vi "Read TDMS File.vi"(8 "error in (no error)":errorcluster, 11 "Path":path) -> (0 "error out":errorcluster, 2 "Data":dbl[](array[numeric]))   [LabVIEW 2022 SP3]
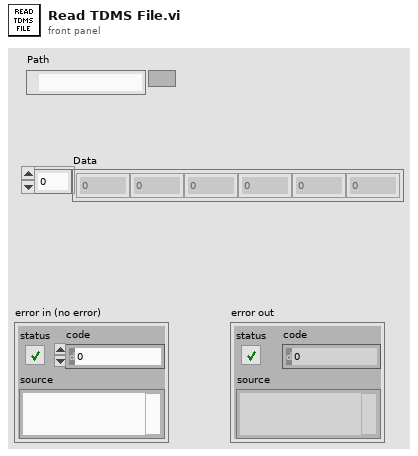
[diagram p1: front panel]
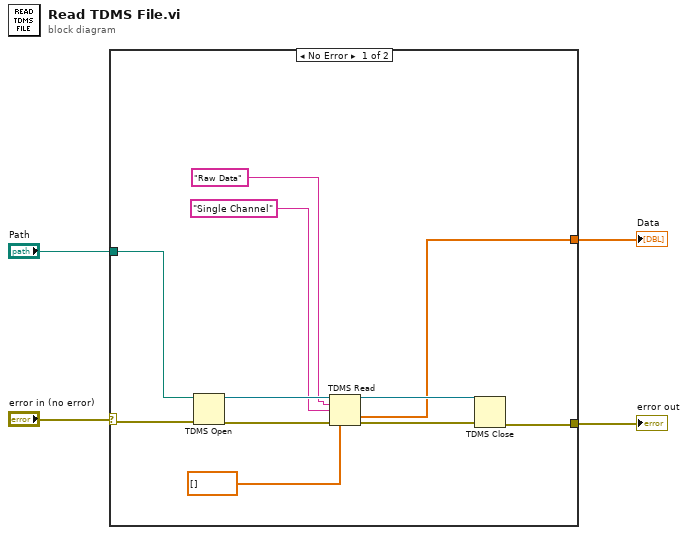
[diagram p0: block diagram]
diagram:
  n1 = case shown="No Error" "error in (no error)" {
    selector: "error in (no error)" -> [w15 w16]
    tunnel: [w13 w16] -> w3
    tunnel: "Path" -> [w14 _]
    tunnel: [w5 _] -> w1
    frame No Error {
      n2 = TDMS Open(8:w15, 11:w14) -> (0:w11:errorcluster, 3:w9:refnum<k34>)  [unwired: 5 in]
      n3 = TDMS Read(0:w9, 5:"Raw Data", 7:"Single Channel", 11:w11, 12:dbl[] []) -> (4:w8:refnum<k34>, 10:w5:dbl[], 15:w12:errorcluster)  [unwired: 3 in, 3 out]
      n4 = TDMS Close(8:w12, 11:w8) -> (0:w13:errorcluster)  [unwired: 1 out]
    }
    frame Error {
    }
  }
  "error out" <- w3
  "Data" <- w1
